vi "Draw Point.vi"(6 "Draw Para":T1={"fill?(F)"=TRUE, "color(black)"=0, "pen"={"Width"=1, "Style"=enum."Solid"}}, 8 "错误输入":errorcluster, 9 "radius":i16 caption="半径", 10 "Center":T2, 11 "Pic in":picture) -> (0 "错误输出":errorcluster, 3 "Pic out":picture)   [LabVIEW 2011, in "Basic Shape.lvlib"]
uses:
  Basic Shape.lvlib
  Point Custom Control.ctl
  Draw Para Custom Control.ctl
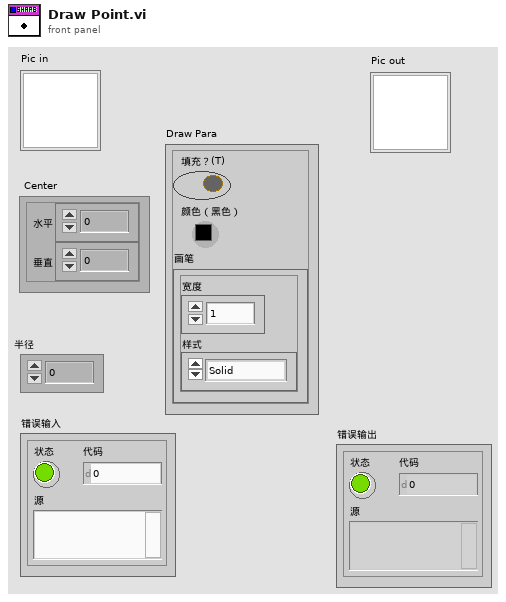
[diagram p1: front panel]
types:
  T1 = typedef "Basic Shape.lvlib/Draw Para Custom Control.ctl" = cluster{"fill?(F)":bool, "color(black)":u32, "pen":cluster{"Width":u16, "Style":enum32{"Solid", "Dash", "Dot", "DashDot", "DashDotDot"}}}
  T2 = typedef "Basic Shape.lvlib/Point Custom Control.ctl" = cluster{"horizontal":i16, "vertical":i16}
  T3 = cluster{"Width":u16, "Style":enum32{"Solid", "Dash", "Dot", "DashDot", "DashDotDot"}}
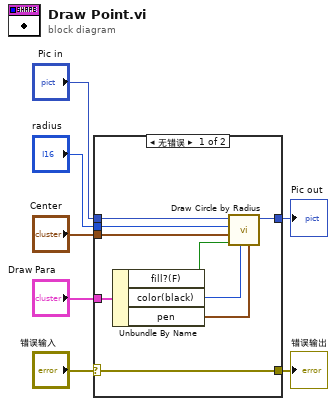
[diagram p0: block diagram]
diagram:
  n1 = case shown="无错误" "错误输入" {
    selector: "错误输入" -> [w16 w18]
    tunnel: [w16 w18] -> w6
    tunnel: "Pic in" -> [w11 w17]
    tunnel: "Center" -> [w9 _]
    tunnel: "Draw Para" -> [w15 _]
    tunnel: [w10 w17] -> w2
    tunnel: "radius" -> [w8 _]
    frame No Error {
      n2 = Unbundle By Name(w15) -> ("fill?(F)"=w14:bool, "color(black)"=w13:u32, "pen"=w12:T3)
      n3 = call <vilib>:"Draw Circle by Radius.vi"("pen"=w12, "color(black)"=w13, "fill?(F)"=w14, "pixel center"=w9, "radius"=w8, "picture"=w11) -> ("new picture"=w10:picture)  [unwired: 5 in]
    }
    frame Error {
    }
  }
  "错误输出" <- w6
  "Pic out" <- w2
